vi "Check Parameter.vi"(6 "Options in":T1={"DbType"=-1, "Direction"=-1, "Size"=-1, "Precision"=255, "Scale"=255} {"Direction" items=["Input"=1, "Output"=2, "InputOutput"=3, "ReturnValue"=6]; "DbType" items=["AnsiString"=0, "Binary"=1, "Byte"=2, "Boolean"=3, "Currency"=4, "Date"=5, "DateTime"=6, "Decimal"=7, "Double"=8, "Guid"=9, "Int16"=10, "Int32"=11, "Int64"=12, "Object"=13, "SByte"=14, "Single"=15, "String"=16, "Time"=17, "UInt16"=18, "UInt32"=19, "UInt64"=20, "VarNumeric"=21, "AnsiStringFixedLength"=22, "StringFixedLength"=23, "Xml"=25, "DateTime2"=26, "DateTimeOffset"=27]}, 8 "error in (no error)":errorcluster, 9 "value in":variant, 10 "name in":string, 11 "PostgresqlConnection in":refnum<class "DBC.lvclass">) -> (0 "error out":errorcluster, 1 "value out":variant, 2 "name out":string, 3 "PostgresqlConnection out":refnum<class "DBC.lvclass">, 4 "Options out":T1={"DbType"=-1, "Direction"=-1, "Size"=-1, "Precision"=255, "Scale"=255} {"Direction" items=["Input"=1, "Output"=2, "InputOutput"=3, "ReturnValue"=6]; "DbType" items=["AnsiString"=0, "Binary"=1, "Byte"=2, "Boolean"=3, "Currency"=4, "Date"=5, "DateTime"=6, "Decimal"=7, "Double"=8, "Guid"=9, "Int16"=10, "Int32"=11, "Int64"=12, "Object"=13, "SByte"=14, "Single"=15, "String"=16, "Time"=17, "UInt16"=18, "UInt32"=19, "UInt64"=20, "VarNumeric"=21, "AnsiStringFixedLength"=22, "StringFixedLength"=23, "Xml"=25, "DateTime2"=26, "DateTimeOffset"=27]})   [LabVIEW 2020, in "ORM_DBC_Npgsql.lvlib" / "DBC.lvclass"]
uses:
  DBC.lvclass
  <vilib>/Viviota/shared/ORM.lvlibp/ORM/DbConnection/DbConnection.lvclass
  <vilib>/regexp/Match Regular Expression.xnode
  <vilib>/JDP Science/JSONtext/JSONtext.lvlib
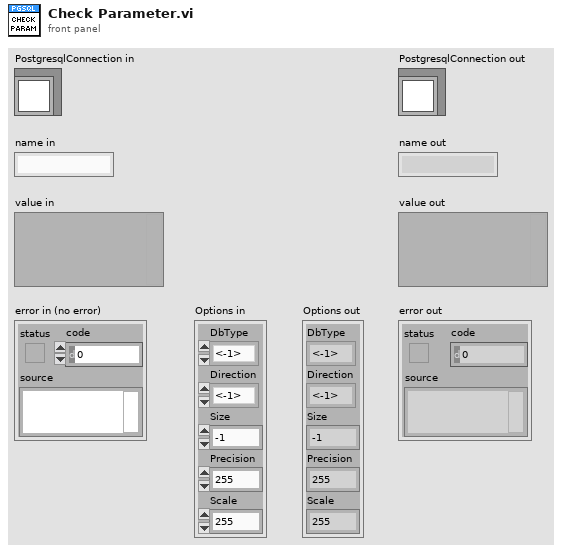
[diagram p1: front panel]
types:
  T1 = cluster{"DbType":i32, "Direction":i32, "Size":i32, "Precision":u8, "Scale":u8}
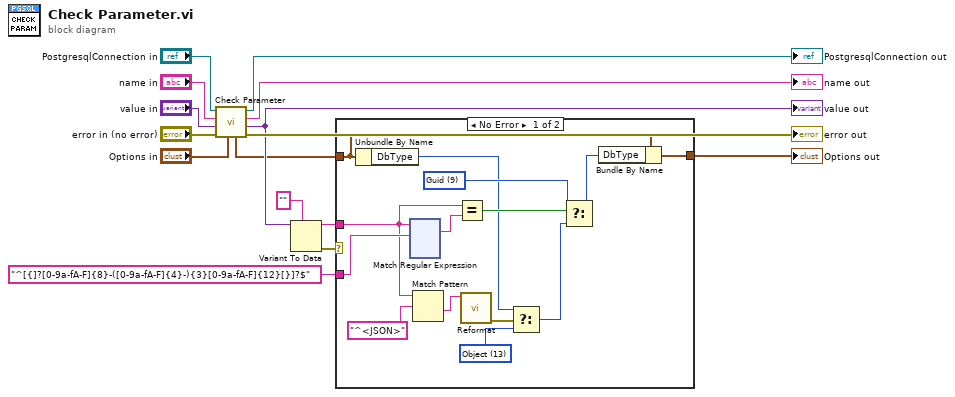
[diagram p0: block diagram]
diagram:
  n1 = call-parent "Check Parameter.vi"("Options in"="Options in", "error in (no error)"="error in (no error)", "value in"="value in", "name in"="name in", "DbConnection in"="PostgresqlConnection in") -> ("error out"=→"error out":errorcluster, "value out"=w8:variant, "name out"=→"name out":string, "DbConnection out"=→"PostgresqlConnection out":refnum<class "DBC.lvclass">, "Options out"=w3:T1)  [unwired: 2 in]
  "value out" <- w8
  n2 = Variant To Data(type="", Variant=w8) -> (data=w5:string, error out=w6:errorcluster)  [unwired: 1 in]
  n3 = case shown="No Error" w6 {
    tunnel: w5 -> [w16 _]
    tunnel: "^[{]?[0-9a-fA-F]{8}-([0-9a-fA-F]{4}-){3}[0-9a-fA-F]{12}[}]?$" -> [w19 _]
    tunnel: w3 -> [w25 w144]
    tunnel: [w24 w144] -> w2
    frame No Error {
      w22 = 13 items=["AnsiString"=0, "Binary"=1, "Byte"=2, "Boolean"=3, "Currency"=4, "Date"=5, "DateTime"=6, "Decimal"=7, "Double"=8, "Guid"=9, "Int16"=10, "Int32"=11, "Int64"=12, "Object"=13, "SByte"=14, "Single"=15, "String"=16, "Time"=17, "UInt16"=18, "UInt32"=19, "UInt64"=20, "VarNumeric"=21, "AnsiStringFixedLength"=22, "StringFixedLength"=23, "Xml"=25, "DateTime2"=26, "DateTimeOffset"=27] ("DbType")
      w27 = 9 items=["AnsiString"=0, "Binary"=1, "Byte"=2, "Boolean"=3, "Currency"=4, "Date"=5, "DateTime"=6, "Decimal"=7, "Double"=8, "Guid"=9, "Int16"=10, "Int32"=11, "Int64"=12, "Object"=13, "SByte"=14, "Single"=15, "String"=16, "Time"=17, "UInt16"=18, "UInt32"=19, "UInt64"=20, "VarNumeric"=21, "AnsiStringFixedLength"=22, "StringFixedLength"=23, "Xml"=25, "DateTime2"=26, "DateTimeOffset"=27] ("DbType")
      n4 = Unbundle By Name(w25) -> ("DbType"=w18:i32)
      n5 = xnode "Match Regular Expression"("input string"=w16, "regular expression"=w19) -> ("whole match"=w29:string)  [unwired: 4 in, 4 out]
      n6 = Match Pattern(string=w16, regular expression="^<JSON>") -> (after substring=w20:string)  [unwired: 1 in, 3 out]
      n7 = Equal?(x=w16, y=w29) -> (x = y?=w28:bool)
      n8 = call <vilib>:"Reformat.vi"("JSON"=w20) -> ("error out"=w23:errorcluster)  [unwired: 7 in, 3 out]
      n9 = Select(t=w18, s=w23, f=w22) -> (s? t:f=w17:i32)
      n10 = Select(t=w27, s=w28, f=w17) -> (s? t:f=w26:i32)
      n11 = Bundle By Name(cluster=w25, "DbType"=w26) -> (w24:T1)
    }
    frame Error {
    }
  }
  "Options out" <- w2
